vi "Get Protocol.vi"(8 "Error In":errorcluster, 11 "Instrument Addon Refnum In":T1 format="%.0x") -> (0 "Error Out":errorcluster, 2 "Protocol":refnum<class "Protocol Parent.lvclass">, 3 "Instrument Addon Refnum Out":T1=18446744073709551615 format="%.0x")   [LabVIEW 2018, in "Instrument Addon Scripting API.lvlib"]
doc: "Outputs the Protocol object corresponding to the provided Instrument Addon Custom Device.\n\nThe output Protocol object can be type-casted to an instance of the following classes: TCP.lvclass, UDP.lvclass, VISA.lvclass, RS-xxx.lvclass, AK TCP.lvclass, AK RS-xxx.lvclass, RS-xxx to GPIB ConvBox.lvclass"
uses:
  Instrument Addon Scripting API.lvlib
  <vilib>/NI Veristand/Custom Device API/Custom Device Item Ref.ctl
  Addon/Support Libraries/Protocols.lvlibp/Protocol Parent/Protocol Parent.lvclass
  Addon/Addon Shared/Types/FG Control.ctl
  Addon/Support Libraries/Protocols.lvlibp/RS-xxx/RS-xxx.lvclass
  C:/Users/nitest/Git/NI VS Instrument Addon Fork/Source/Addon/Support Libraries/Protocols.lvlibp/Protocol Parent/Protocol Parent.lvclass
  Addon/Support Libraries/Protocols.lvlibp/AK RS-xxx/AK RS-xxx.lvclass
  C:/Users/nitest/Git/NI VS Instrument Addon Fork/Source/Addon/Support Libraries/Protocols.lvlibp/RS-xxx/RS-xxx.lvclass
  Addon/Support Libraries/Protocols.lvlibp/VISA/VISA.lvclass
  Addon/Support Libraries/Protocols.lvlibp/AK TCP/AK TCP.lvclass
  C:/Users/nitest/Git/NI VS Instrument Addon Fork/Source/Addon/Support Libraries/Protocols.lvlibp/TCP/TCP.lvclass
  Addon/Support Libraries/Protocols.lvlibp/TCP/TCP.lvclass
  Addon/Support Libraries/Protocols.lvlibp/UDP/UDP.lvclass
  Addon/Support Libraries/Protocols.lvlibp/RS-xxx to GPIB ConvBox/RS-xxx to GPIB ConvBox.lvclass
  Addon/Addon Shared/SubVIs/Constants.vi
  <vilib>/NI/NI VeriStand Advanced SysDef API/SysDef API/SysDef.Property.Get.vi
  <vilib>/NI/NI VeriStand Advanced SysDef API/_SubVIs/SysDef.Property.Get.String.vi
  <vilib>/NI/NI VeriStand Advanced SysDef API/SysDef API/SysDef.Property.Set.vi
  <vilib>/NI/NI VeriStand Advanced SysDef API/_SubVIs/SysDef.Property.Set.String.vi
  <vilib>/Utility/LVClass/Get LV Class Default Value.vi
  <vilib>/NI Veristand/Custom Device API/NI VeriStand - Get Item Property.vi
  <vilib>/NI Veristand/Custom Device API/Get Item Property (String).vi
  <vilib>/NI Veristand/Custom Device API/Get Item Property (U32).vi
  <vilib>/NI Veristand/Custom Device API/Get Item Property (Boolean).vi
  <vilib>/NI Veristand/Custom Device API/NI VeriStand - Set Item Property.vi
  <vilib>/NI Veristand/Custom Device API/Set Item Property (String).vi
  <vilib>/NI Veristand/Custom Device API/Set Item Property (U32).vi
  <vilib>/NI Veristand/Custom Device API/Set Item Property (Boolean).vi
  Addon/Support Libraries/Protocols.lvlibp/RS-xxx/Data Access/Write PortSettings.vi
  Addon/Support Libraries/Protocols.lvlibp/VISA/Data Access/Write VISA Resource.vi
  Addon/Support Libraries/Protocols.lvlibp/VISA/Data Access/Write Enable Termination Character.vi
  Addon/Support Libraries/Protocols.lvlibp/VISA/Data Access/Write Termination Character.vi
  Addon/Support Libraries/Protocols.lvlibp/VISA/Data Access/Write Timeout.vi
  Addon/Support Libraries/Protocols.lvlibp/VISA/Data Access/Write Append Write Termination Character.vi
  Addon/Support Libraries/Protocols.lvlibp/TCP/Data Access/Write IP Address.vi
  Addon/Support Libraries/Protocols.lvlibp/TCP/Data Access/Write Port.vi
  Addon/Support Libraries/Protocols.lvlibp/UDP/Data Access/Write Local IP Address.vi
  Addon/Support Libraries/Protocols.lvlibp/UDP/Data Access/Write Local Port.vi
  Addon/Support Libraries/Protocols.lvlibp/UDP/Data Access/Write Target IP Address.vi
  Addon/Support Libraries/Protocols.lvlibp/UDP/Data Access/Write Target Port.vi
  Addon/Support Libraries/Protocols.lvlibp/RS-xxx to GPIB ConvBox/Data Access/Write Port.vi
  Addon/Support Libraries/Protocols.lvlibp/RS-xxx to GPIB ConvBox/Data Access/Write ConvBox Address.vi
  Addon/Support Libraries/Protocols.lvlibp/RS-xxx to GPIB ConvBox/Data Access/Write Assert Ren with IFC.vi
  Addon/Support Libraries/Protocols.lvlibp/RS-xxx to GPIB ConvBox/Data Access/Write System controller.vi
  Addon/Support Libraries/Protocols.lvlibp/RS-xxx to GPIB ConvBox/Data Access/Write IST bit sense.vi
  Addon/Support Libraries/Protocols.lvlibp/RS-xxx to GPIB ConvBox/Data Access/Write GPIB Address.vi
  Addon/Addon Shared/Instrument Addon Shared.lvlib
  <vilib>/NI Veristand/Custom Device API/Custom Device API.lvlib
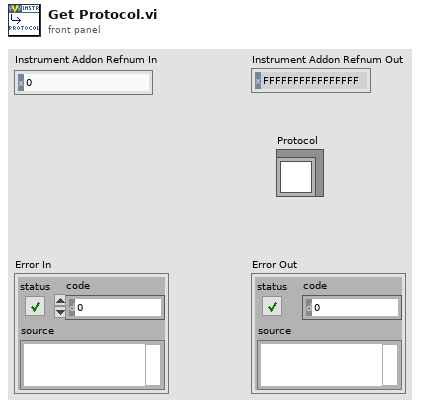
[diagram p1: front panel]
types:
  T1 = typedef "Custom Device API.lvlib/Custom Device Item Ref.ctl" = u64
  T2 = typedef "Instrument Addon Shared.lvlib/FG Control.ctl" = enum16{"Get", "Set"}
  T3 = cluster{"Port":string, "Baud Rate":u32, "Data Bits":u16, "Parity":enum16{"None", "Odd", "Even", "Mark", "Space"}, "Stop Bits":u16, "Flow Control":u16, "XON":enum16{"NUL", "SOH", "STX", "ETX", "EOT", "ENQ", "ACK", "BEL", "BS", "HT", "LF", "VT", "FF", "CR", "SO", "SI", "DLE", "DC1", "DC2", "DC3", "DC4", "NAK", "SYN", "ETB", "CAN", "EM", "SUB", "ESC", "FS", "GS", "RS", "US", "SP", "!", "\"", "#", "$", "%", "&", "'", "(", ")", "*", "+", ",", "- (-)", ".", "/", "0", "1", "2", "3", "4", "5", "6", "7", "8", "9", ":", ";", "<", "=", ">", "?", "@", "A", "B", "C", "D", "E", "F", "G", "H", "I", "J", "K", "L", "M", "N", "O", "P", "Q", "R", "S", "T", "U", "V", "W", "X", "Y", "Z", "[", "\\", "]", "^", "_", "`", "a", "b", "c", "d", "e", "f", "g", "h", "i", "j", "k", "l", "m", "n", "o", "p", "q", "r", "s", "t", "u", "v", "w", "x", "y", "z", "{", "|", "}", "~"}, "XOFF":enum16{"NUL", "SOH", "STX", "ETX", "EOT", "ENQ", "ACK", "BEL", "BS", "HT", "LF", "VT", "FF", "CR", "SO", "SI", "DLE", "DC1", "DC2", "DC3", "DC4", "NAK", "SYN", "ETB", "CAN", "EM", "SUB", "ESC", "FS", "GS", "RS", "US", "SP", "!", "\"", "#", "$", "%", "&", "'", "(", ")", "*", "+", ",", "- (-)", ".", "/", "0", "1", "2", "3", "4", "5", "6", "7", "8", "9", ":", ";", "<", "=", ">", "?", "@", "A", "B", "C", "D", "E", "F", "G", "H", "I", "J", "K", "L", "M", "N", "O", "P", "Q", "R", "S", "T", "U", "V", "W", "X", "Y", "Z", "[", "\\", "]", "^", "_", "`", "a", "b", "c", "d", "e", "f", "g", "h", "i", "j", "k", "l", "m", "n", "o", "p", "q", "r", "s", "t", "u", "v", "w", "x", "y", "z", "{", "|", "}", "~"}, "End Read on Termination Character":bool, "End Write on Termination Character":bool, "Termination Character":u8}
  T4 = typedef "Protocols.lvlibp/Protocol Parent.lvclass/Base Protocol Type.ctl" = enum16{"RS-XXX", "VISA", "TCPIP", "UDP", "GPIB ConvBox"}
  T5 = typedef "Instrument Addon Shared.lvlib/RSXXX Port Settings.ctl" = cluster{"Port":string, "Baud Rate":u32, "Data Bits":u16, "Parity":enum16{"None", "Odd", "Even", "Mark", "Space"}, "Stop Bits":u16, "Flow Control":u16, "XON":enum16{"NUL", "SOH", "STX", "ETX", "EOT", "ENQ", "ACK", "BEL", "BS", "HT", "LF", "VT", "FF", "CR", "SO", "SI", "DLE", "DC1", "DC2", "DC3", "DC4", "NAK", "SYN", "ETB", "CAN", "EM", "SUB", "ESC", "FS", "GS", "RS", "US", "SP", "!", "\"", "#", "$", "%", "&", "'", "(", ")", "*", "+", ",", "- (-)", ".", "/", "0", "1", "2", "3", "4", "5", "6", "7", "8", "9", ":", ";", "<", "=", ">", "?", "@", "A", "B", "C", "D", "E", "F", "G", "H", "I", "J", "K", "L", "M", "N", "O", "P", "Q", "R", "S", "T", "U", "V", "W", "X", "Y", "Z", "[", "\\", "]", "^", "_", "`", "a", "b", "c", "d", "e", "f", "g", "h", "i", "j", "k", "l", "m", "n", "o", "p", "q", "r", "s", "t", "u", "v", "w", "x", "y", "z", "{", "|", "}", "~"}, "XOFF":enum16{"NUL", "SOH", "STX", "ETX", "EOT", "ENQ", "ACK", "BEL", "BS", "HT", "LF", "VT", "FF", "CR", "SO", "SI", "DLE", "DC1", "DC2", "DC3", "DC4", "NAK", "SYN", "ETB", "CAN", "EM", "SUB", "ESC", "FS", "GS", "RS", "US", "SP", "!", "\"", "#", "$", "%", "&", "'", "(", ")", "*", "+", ",", "- (-)", ".", "/", "0", "1", "2", "3", "4", "5", "6", "7", "8", "9", ":", ";", "<", "=", ">", "?", "@", "A", "B", "C", "D", "E", "F", "G", "H", "I", "J", "K", "L", "M", "N", "O", "P", "Q", "R", "S", "T", "U", "V", "W", "X", "Y", "Z", "[", "\\", "]", "^", "_", "`", "a", "b", "c", "d", "e", "f", "g", "h", "i", "j", "k", "l", "m", "n", "o", "p", "q", "r", "s", "t", "u", "v", "w", "x", "y", "z", "{", "|", "}", "~"}, "End Read on Termination Character":bool, "End Write on Termination Character":bool, "Termination Character":u8}
  T6 = enum16{"NUL", "SOH", "STX", "ETX", "EOT", "ENQ", "ACK", "BEL", "BS", "HT", "LF", "VT", "FF", "CR", "SO", "SI", "DLE", "DC1", "DC2", "DC3", "DC4", "NAK", "SYN", "ETB", "CAN", "EM", "SUB", "ESC", "FS", "GS", "RS", "US", "SP", "!", "\"", "#", "$", "%", "&", "'", "(", ")", "*", "+", ",", "- (-)", ".", "/", "0", "1", "2", "3", "4", "5", "6", "7", "8", "9", ":", ";", "<", "=", ">", "?", "@", "A", "B", "C", "D", "E", "F", "G", "H", "I", "J", "K", "L", "M", "N", "O", "P", "Q", "R", "S", "T", "U", "V", "W", "X", "Y", "Z", "[", "\\", "]", "^", "_", "`", "a", "b", "c", "d", "e", "f", "g", "h", "i", "j", "k", "l", "m", "n", "o", "p", "q", "r", "s", "t", "u", "v", "w", "x", "y", "z", "{", "|", "}", "~"}
  T7 = typedef "Instrument Addon Shared.lvlib/VISA Settings.ctl" = cluster{"VISA Resource":string, "Enable Termination Character":bool, "Termination Character":u8, "Timeout":u32, "Append Write Termination Character":bool}
  T8 = typedef "Instrument Addon Shared.lvlib/TCPIP Settings.ctl" = cluster{"IP Address":string, "Port":u16}
  T9 = typedef "Instrument Addon Shared.lvlib/UDP Settings.ctl" = cluster{"Local IP Address":string, "Local Port":u16, "Target IP Address":string, "Target Port":u16}
  T10 = typedef "Instrument Addon Shared.lvlib/GPIB ConvBox Settings.ctl" = cluster{"Port":string, "ConvBox Address":string, "Assert Ren with IFC":bool, "System controller":bool, "IST bit sense":bool, "GPIB Address":string}
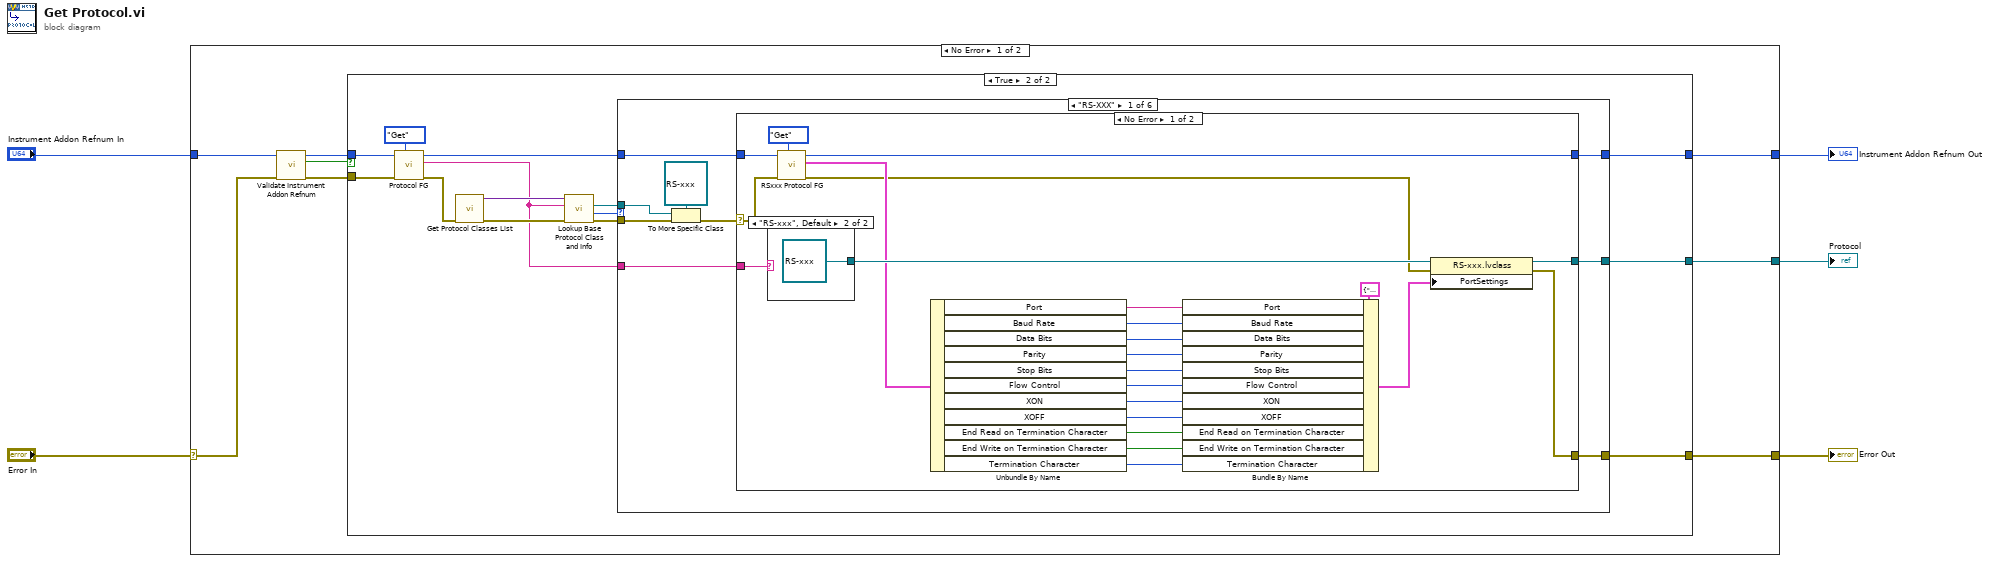
[diagram p0: block diagram]
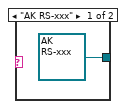
[diagram p3: hidden frame]
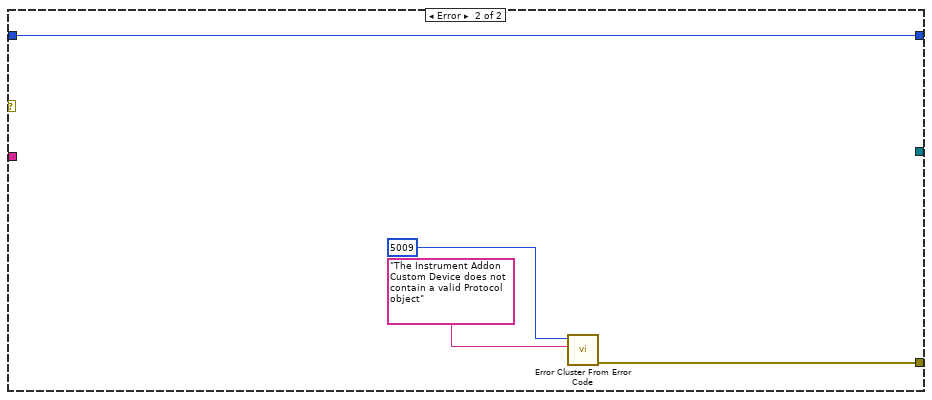
[diagram p4: hidden frame]
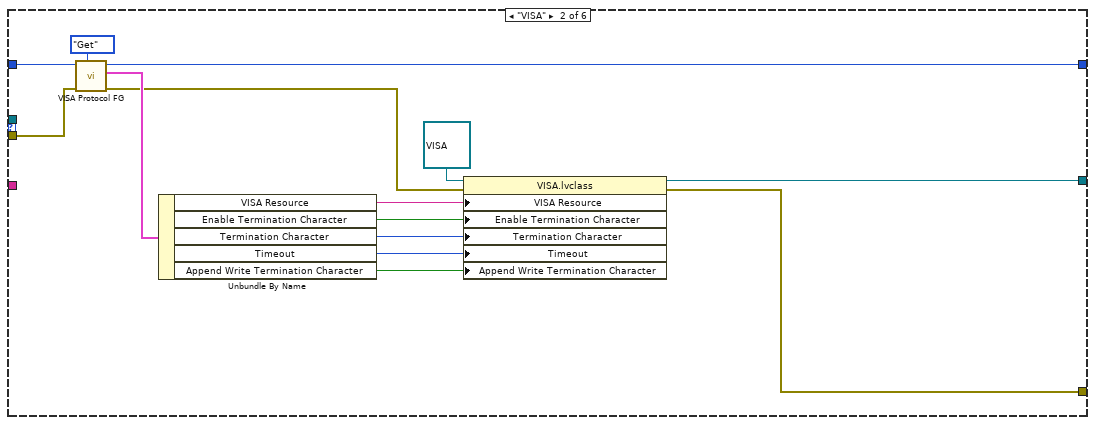
[diagram p5: hidden frame]
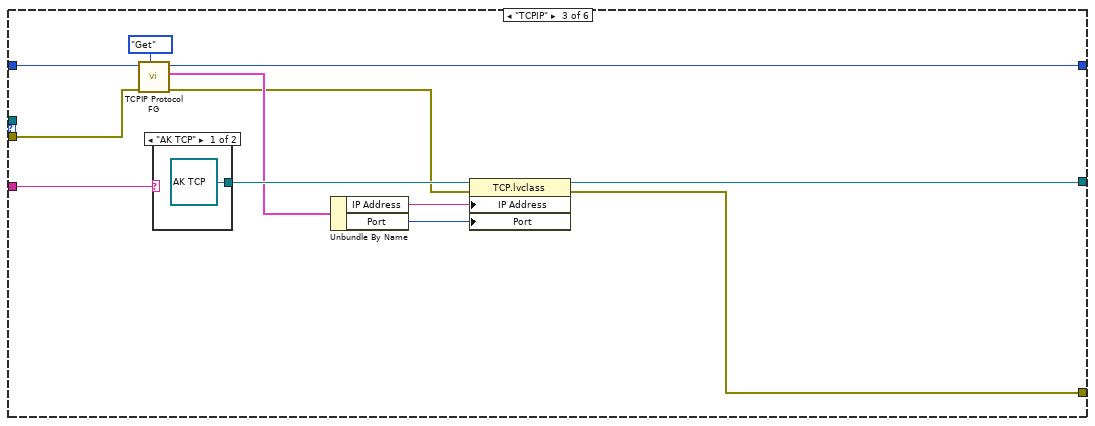
[diagram p6: hidden frame]
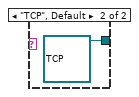
[diagram p7: hidden frame]
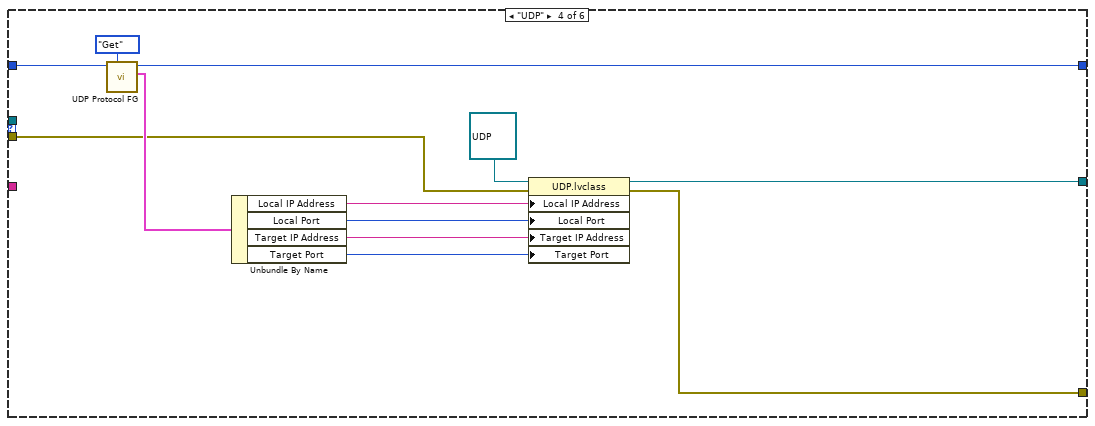
[diagram p8: hidden frame]
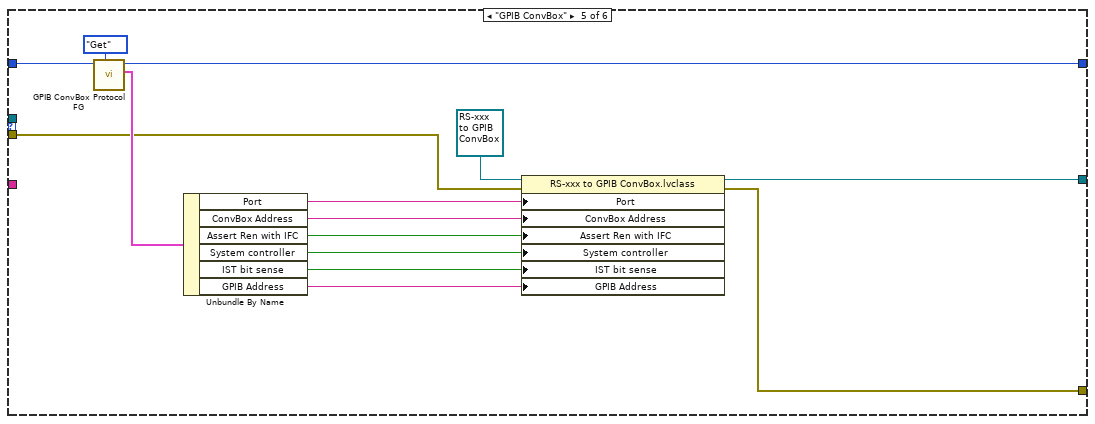
[diagram p9: hidden frame]
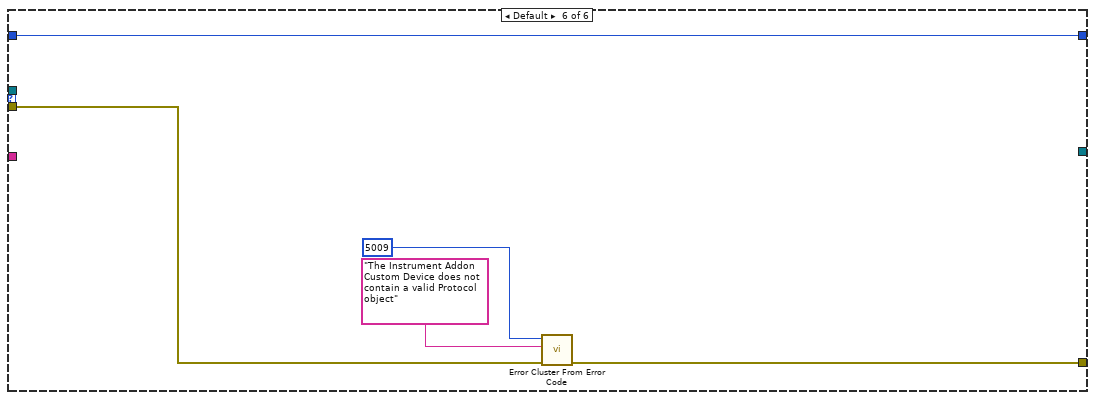
[diagram p10: hidden frame]
diagram:
  n1 = case shown="No Error" "Error In" {
    selector: "Error In" -> [w12 w128]
    tunnel: "Instrument Addon Refnum In" -> [w13 w127]
    tunnel: [w9 w128] -> w4
    tunnel: [w8 w127] -> w2
    tunnel: [w6 _] -> w1
    frame No Error {
      n2 = call "Validate Instrument Addon Refnum.vi"("Error In"=w12, "Refnum In"=w13) -> ("Error Out"=w7:errorcluster, "Is Instrument Addon?"=w10:bool, "Refnum Out"=w11:T1)  [unwired: 7 in]
      n3 = case shown="True" w10 {
        tunnel: w11 -> [w15 w28]
        tunnel: [w14 w17] -> w9
        tunnel: [w15 w18] -> w8
        tunnel: w7 -> [w14 w27]
        tunnel: [_ w19] -> w6
        frame False {
        }
        frame True {
          n4 = call "Protocol FG.vi"("Action"=FG_Control."Get", "error in (no error)"=w27, "Device Item Ref in"=w28) -> ("error out"=w26:errorcluster, "Protocol out"=w16:string, "Item Ref out"=w23:T1)  [unwired: 6 in]
          n5 = call "Get Protocol Classes List.vi"("error in (no error)"=w26) -> ("error out"=w25:errorcluster, "Class Lookup"=w24:variant)  [unwired: 9 in]
          n6 = call "Lookup Base Protocol Class and Info.vi"("error in (no error)"=w25, "Protocol in"=w16, "Class Lookup"=w24) -> ("error out"=w21:errorcluster, "Protocol out"=w22:T4, "Protocol Parent out"=w20:refnum<class "Protocol Parent.lvclass">)  [unwired: 4 in, 2 out]
          n7 = case shown="\"RS-XXX\"" w22 {
            tunnel: w23 -> [w37 w80 w90 w105 w119 w126]
            tunnel: w21 -> [w32 w79 w89 w96 w109 w123]
            tunnel: w20 -> [w33 _ _ _ _ _]
            tunnel: [w35 w72 w84 w98 w110 _] -> w19
            tunnel: [w36 w69 w83 w99 w111 w126] -> w18
            tunnel: [w34 w68 w82 w97 w108 w122] -> w17
            tunnel: w16 -> [w38 _ w93 _ _ _]
            frame "RS-XXX" {
              n8 = To More Specific Class(target class=refnum<class "RS-xxx.lvclass"> refnum ("Protocols.lvlibp:RS-xxx.lvclass"), reference=w33, error in=w32) -> (error out=w31:errorcluster)  [unwired: 1 out]
              n9 = case shown="No Error" w31 {
                selector: w31 -> [w39 _]
                tunnel: w38 -> [w61 _]
                tunnel: w37 -> [w59 w64]
                tunnel: [w43 w64] -> w36
                tunnel: [w42 _] -> w35
                tunnel: [w40 w65] -> w34
                frame No Error {
                  n10 = case shown="\"RS-xxx\", Default" w61 {
                    tunnel: [refnum<class "AK RS-xxx.lvclass"> refnum ("Protocols.lvlibp:AK RS-xxx.lvclass") refnum<class "RS-xxx.lvclass"> refnum ("Protocols.lvlibp:RS-xxx.lvclass")] -> w58
                    frame "AK RS-xxx" {
                    }
                    frame "RS-xxx", Default {
                    }
                  }
                  n11 = call "RSxxx Protocol FG.vi"("Action"=FG_Control."Get", "error in (no error)"=w39, "Device Item Ref in"=w59) -> ("error out"=w41:errorcluster, "Serial Config"=w56:T5, "Item Ref out"=w43:T1)  [unwired: 6 in]
                  n12 = Unbundle By Name(w56) -> ("Port"=w55:string, "Baud Rate"=w54:u32, "Data Bits"=w53:u16, "Parity"=w52:enum16{"None", "Odd", "Even", "Mark", "Space"}, "Stop Bits"=w51:u16, "Flow Control"=w50:u16, "XON"=w49:T6, "XOFF"=w48:T6, "End Read on Termination Character"=w47:bool, "End Write on Termination Character"=w46:bool, "Termination Character"=w45:u8)
                  n13 = Bundle By Name(cluster=T3 {"Port"="COM1", "Baud Rate"=9600, "Data Bits"=8, "Parity"=enum."None", "Stop Bits"=10, "Flow Control"=0, "XON"=enum."DC1", "XOFF"=enum."DC3", "End Read on Termination Character"=TRUE, "End Write on Termination Character"=TRUE, "Termination Character"=10} ("PortSettings"), "Port"=w55, "Baud Rate"=w54, "Data Bits"=w53, "Parity"=w52, "Stop Bits"=w51, "Flow Control"=w50, "XON"=w49, "XOFF"=w48, "End Read on Termination Character"=w47, "End Write on Termination Character"=w46, "Termination Character"=w45) -> (w44:T3)
                  n14 = property class="RS-xxx.lvclass"(reference=w58, error in=w41, "PortSettings"=w44) -> (reference out=w42:refnum<class "RS-xxx.lvclass">, error out=w40:errorcluster)
                }
                frame Error {
                  n15 = call <vilib>:"Error Cluster From Error Code.vi"("error message (\"\")"="The Instrument Addon Custom Device does not contain a valid Protocol object" ("error message (\"\")"), "error code (0)"=5009) -> ("error out"=w65:errorcluster)  [unwired: 7 in]
                }
              }
            }
            frame "VISA" {
              n16 = call "VISA Protocol FG.vi"("Action"=FG_Control."Get", "error in (no error)"=w79, "Device Item Ref in"=w80) -> ("error out"=w70:errorcluster, "VISA Config"=w78:T7, "Item Ref out"=w69:T1)  [unwired: 6 in]
              n17 = Unbundle By Name(w78) -> ("VISA Resource"=w77:string, "Enable Termination Character"=w76:bool, "Termination Character"=w75:u8, "Timeout"=w74:u32, "Append Write Termination Character"=w73:bool)
              n18 = property class="VISA.lvclass"(reference=refnum<class "VISA.lvclass"> refnum ("Protocols.lvlibp:VISA.lvclass"), error in=w70, "VISA Resource"=w77, "Enable Termination Character"=w76, "Termination Character"=w75, "Timeout"=w74, "Append Write Termination Character"=w73) -> (reference out=w72:refnum<class "VISA.lvclass">, error out=w68:errorcluster)
            }
            frame "TCPIP" {
              n19 = call "TCPIP Protocol FG.vi"("Action"=FG_Control."Get", "error in (no error)"=w89, "Device Item Ref in"=w90) -> ("error out"=w85:errorcluster, "TCP/IP Config"=w88:T8, "Item Ref out"=w83:T1)  [unwired: 6 in]
              n20 = case shown="\"AK TCP\"" w93 {
                tunnel: [refnum<class "AK TCP.lvclass"> refnum ("Protocols.lvlibp:AK TCP.lvclass") refnum<class "TCP.lvclass"> refnum ("Protocols.lvlibp:TCP.lvclass")] -> w92
                frame "AK TCP" {
                }
                frame "TCP", Default {
                }
              }
              n21 = Unbundle By Name(w88) -> ("IP Address"=w87:string, "Port"=w86:u16)
              n22 = property class="TCP.lvclass"(reference=w92, error in=w85, "IP Address"=w87, "Port"=w86) -> (reference out=w84:refnum<class "TCP.lvclass">, error out=w82:errorcluster)
            }
            frame "UDP" {
              n23 = call "UDP Protocol FG.vi"("Action"=FG_Control."Get", "Device Item Ref in"=w105) -> ("UDP Config"=w104:T9, "Item Ref out"=w99:T1)  [unwired: 7 in, 1 out]
              n24 = Unbundle By Name(w104) -> ("Local IP Address"=w103:string, "Local Port"=w102:u16, "Target IP Address"=w101:string, "Target Port"=w100:u16)
              n25 = property class="UDP.lvclass"(reference=refnum<class "UDP.lvclass"> refnum ("Protocols.lvlibp:UDP.lvclass"), error in=w96, "Local IP Address"=w103, "Local Port"=w102, "Target IP Address"=w101, "Target Port"=w100) -> (reference out=w98:refnum<class "UDP.lvclass">, error out=w97:errorcluster)
            }
            frame "GPIB ConvBox" {
              n26 = call "GPIB ConvBox Protocol FG.vi"("Action"=FG_Control."Get", "Device Item Ref in"=w119) -> ("GPIB ConvBox Config"=w118:T10, "Item Ref out"=w111:T1)  [unwired: 7 in, 1 out]
              n27 = Unbundle By Name(w118) -> ("Port"=w117:string, "ConvBox Address"=w116:string, "Assert Ren with IFC"=w115:bool, "System controller"=w114:bool, "IST bit sense"=w113:bool, "GPIB Address"=w112:string)
              n28 = property class="RS-xxx to GPIB ConvBox.lvclass"(reference=refnum<class "RS-xxx to GPIB ConvBox.lvclass"> refnum ("Protocols.lvlibp:RS-xxx to GPIB ConvBox.lvclass"), error in=w109, "Port"=w117, "ConvBox Address"=w116, "Assert Ren with IFC"=w115, "System controller"=w114, "IST bit sense"=w113, "GPIB Address"=w112) -> (reference out=w110:refnum<class "RS-xxx to GPIB ConvBox.lvclass">, error out=w108:errorcluster)
            }
            frame Default {
              n29 = call <vilib>:"Error Cluster From Error Code.vi"("error in (no error)"=w123, "error message (\"\")"="The Instrument Addon Custom Device does not contain a valid Protocol object" ("error message (\"\")"), "error code (0)"=5009) -> ("error out"=w122:errorcluster)  [unwired: 6 in]
            }
          }
        }
      }
    }
    frame Error {
    }
  }
  "Error Out" <- w4
  "Instrument Addon Refnum Out" <- w2
  "Protocol" <- w1
